vi "tlc_Load.vi"(8 "error in (no error)":errorcluster, 10 "Path":path) -> (0 "error out":errorcluster)   [LabVIEW 2018]
uses:
  Modules/File/tlc_File_Command Control.ctl
  Controls/tlc_User Interface Data Type.ctl
  Modules/Cue/tlc_Cue_Information Command.ctl
panel:
  # "Input"
  # "Output"
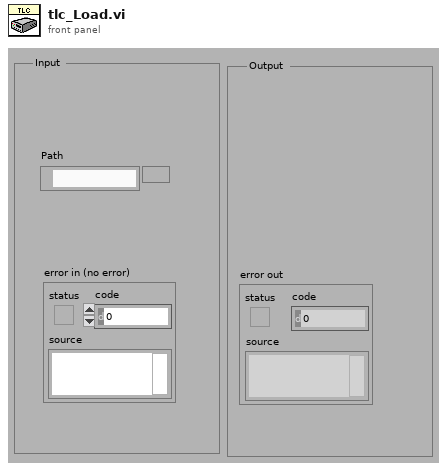
[diagram p1: front panel]
types:
  T1 = typedef "tlc_User Interface Data Type.ctl" = enum16{"Initialize", "Initialize Front Panel", "Update Front Panel Channels", "Select Cue in Cue List", "Enable/Disable Front Panel Controls", "Update Cue List", "Stop"}
  T2 = typedef "tlc_Cue_Information Command.ctl" = enum16{"Add Cue", "Delete Cue", "Get Cue Values", "Set Cue Values", "Swap", "Get Number of Cues", "Initialize", "Get Empty Cue"}
  T3 = typedef "tlc_File_Command Control.ctl" = enum16{"Initialize", "Save Cues", "Load Cues", "Shutdown"}
  T4 = typedef "tlc_Cue_Information.ctl" = cluster{"Cue Name":string, "Wait Time (s)":u32, "Fade Time (s)":u32, "Follow Time (s)":u32, "Channels":T5[][]}
  T5 = typedef "channel.ctl" = cluster{"Intensity":dbl, " Color":u32, "Channel":i32}
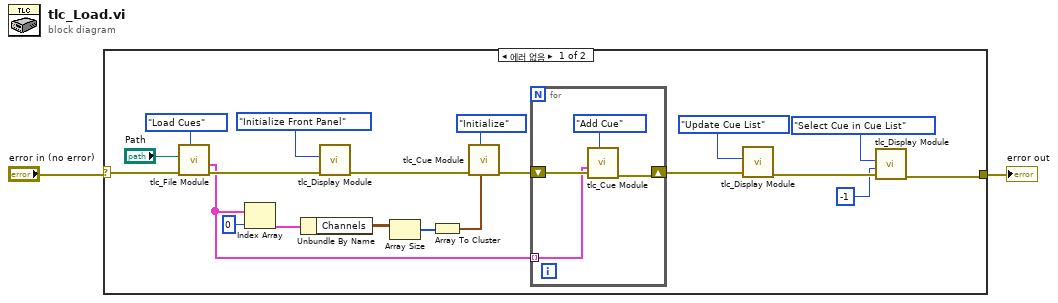
[diagram p0: block diagram]
diagram:
  n1 = case shown="에러 없음" "error in (no error)" {
    selector: "error in (no error)" -> [w22 w27]
    tunnel: [w5 w27] -> w1
    frame No Error {
      n2 = call "tlc_File Module.vi"("Command"=tlc_File_Command_Control."Load Cues", "error in (no error)"=w22, "Path"="Path") -> ("error out"=w19:errorcluster, "Cue Array Output"=w9:T4[])  [unwired: 7 in]
      n3 = Index Array(array=w9, index=0) -> (element=w14:T4)
      n4 = Unbundle By Name(w14) -> ("Channels"=w13:T5[][])
      n5 = call "tlc_Display Module.vi"("error in (no error)"=w19, "Data Type"=tlc_User_Interface_Data_Type."Initialize Front Panel") -> ("error out"=w17:errorcluster)  [unwired: 9 in]
      n6 = Array Size(array=w13) -> (size(s)=w12:i32[])
      n7 = Array To Cluster(array=w12) -> (cluster=w11:cluster{"[0]":i32, "[1]":i32})
      n8 = call "tlc_Cue Module.vi"("Number of Channels"=w11, "Command"=tlc_Cue_Information_Command."Initialize", "error in (no error)"=w17) -> ("error out"=w10:errorcluster)  [unwired: 5 in, 2 out]
      n9 = for {
        shift-right: [w25] -> w8
        shift-left: w10 -> [w26]
        tunnel: w9 -> [w23] mode=indexing
        n10 = call "tlc_Cue Module.vi"("Command"=tlc_Cue_Information_Command."Add Cue", "error in (no error)"=w26, "Cue Input"=w23) -> ("error out"=w25:errorcluster)  [unwired: 5 in, 2 out]
      }
      n11 = call "tlc_Display Module.vi"("error in (no error)"=w8, "Data Type"=tlc_User_Interface_Data_Type."Update Cue List") -> ("error out"=w6:errorcluster)  [unwired: 9 in]
      n12 = call "tlc_Display Module.vi"("error in (no error)"=w6, "Data"=-1, "Data Type"=tlc_User_Interface_Data_Type."Select Cue in Cue List") -> ("error out"=w5:errorcluster)  [unwired: 8 in]
    }
    frame Error {
    }
  }
  "error out" <- w1
